vi "Is Express VI.vi"(8 "error in":errorcluster, 11 "VI Reference":refnum<vi>) -> (0 "error out":errorcluster, 1 "Is Instance":bool, 2 "Is Express VI":bool, 3 "Display Name":string)   [LabVIEW 2020, in "Peek Window.lvlib"]
uses:
  Peek Window.lvlib
  8898ce48-ddb9-4dd9-ab7b-7e2c6aebdd87.vi
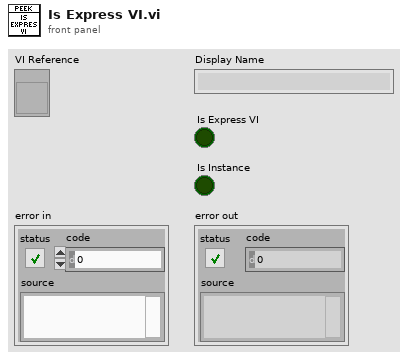
[diagram p1: front panel]
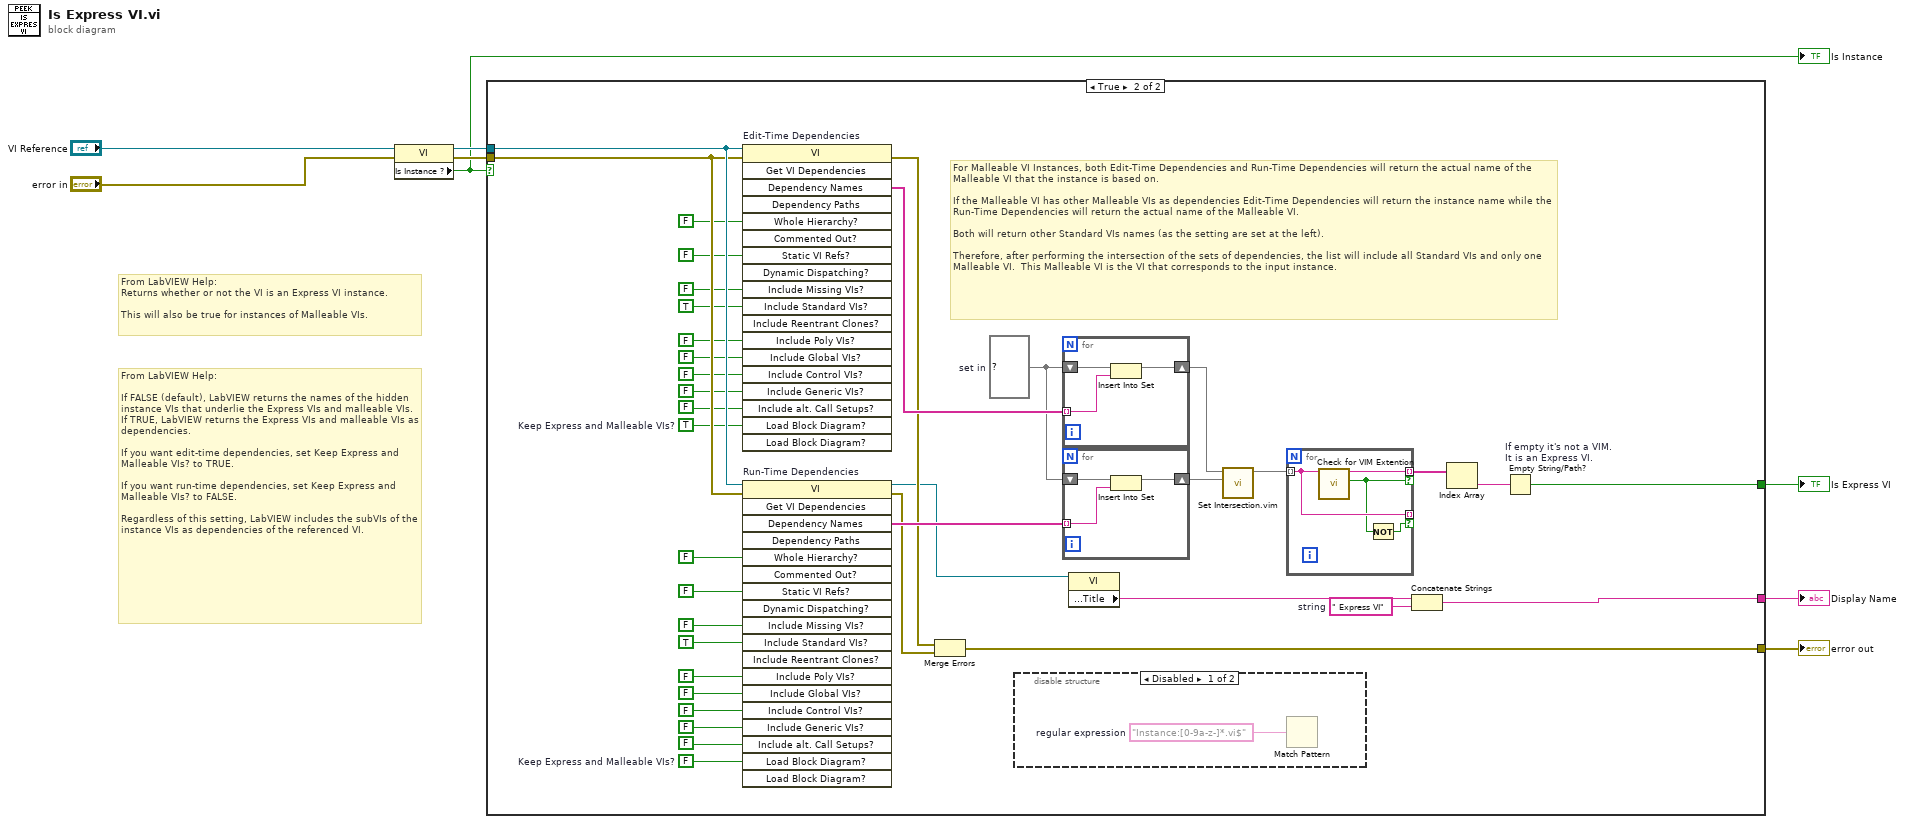
[diagram p0: block diagram]
diagram:
  # "From LabVIEW Help:\nReturns whether or not the VI is an Express VI instance.\n\nThis will also be true for instances of Malleable VIs."
  # "From LabVIEW Help:\n\nIf FALSE (default), LabVIEW returns the names of the hidden instance VIs that underlie the Express VIs and malleable VIs. If TRUE, LabVIEW returns the Express VIs and malleable VIs as dependencies.\n\nIf you want edit-time dependencies, set Keep Express and Malleable VIs? to TRUE. \n\nIf you want run-time dependencies, set Keep Express and Malleable VIs? to FALSE. \n\nRegardless of this setting, LabVIEW includes the subVIs of the instance VIs as dependencies of the referenced VI."
  n1 = property class="VI"(reference="VI Reference", error in="error in") -> (reference out=w8:refnum<vi>, error out=w7:errorcluster, "Is Instance ?"=w3:bool)
  "Is Instance" <- w3
  n2 = case shown="True" w3 {
    tunnel: w8 -> [_ w47]
    tunnel: w7 -> [w9 w45]
    tunnel: [w9 w44] -> w6
    tunnel: [_ w14] -> w2
    tunnel: [_ w11] -> w1
    frame False {
    }
    frame True {
      w10 = " Express VI"  # string
      w19 = set{string} {}  # set in
      w24 = FALSE  # Keep Express and Malleable VIs?
      w43 = TRUE  # Keep Express and Malleable VIs?
      # "For Malleable VI Instances, both Edit-Time Dependencies and Run-Time Dependencies will return the actual name of the Malleable VI that the instance is based on.  \n\nIf the Malleable VI has other Malleable VIs as dependencies Edit-Time Dependencies will return the instance name while the Run-Time Dependencies will return the actual name of the Malleable VI.\n\nBoth will return other Standard VIs names (as the setting are set at the left).\n\nTherefore, after performing the intersection of the sets of dependencies, the list will include all Standard VIs and only one Malleable VI.  This Malleable VI is the VI that corresponds to the input instance."
      n3 = invoke on="Edit-Time Dependencies" class="VI" method="Get VI Dependencies"(reference=w47, error in=w45, "Whole Hierarchy?"=FALSE, "Static VI Refs?"=FALSE, "Include Missing VIs?"=FALSE, "Include Standard VIs?"=TRUE, "Include Poly VIs?"=FALSE, "Include Global VIs?"=FALSE, "Include Control VIs?"=FALSE, "Include Generic VIs?"=FALSE, "Include alt. Call Setups?"=FALSE, "Load Block Diagram?"=w43) -> (error out=w16:errorcluster, "Dependency Names"=w23:string[])  [unwired: 7 in, 17 out]
      n4 = invoke on="Run-Time Dependencies" class="VI" method="Get VI Dependencies"(reference=w47, error in=w45, "Whole Hierarchy?"=FALSE, "Static VI Refs?"=FALSE, "Include Missing VIs?"=FALSE, "Include Standard VIs?"=TRUE, "Include Poly VIs?"=FALSE, "Include Global VIs?"=FALSE, "Include Control VIs?"=FALSE, "Include Generic VIs?"=FALSE, "Include alt. Call Setups?"=FALSE, "Load Block Diagram?"=w24) -> (reference out=w13:refnum<vi>, error out=w15:errorcluster, "Dependency Names"=w18:string[])  [unwired: 7 in, 16 out]
      n5 = Merge Errors(w16, w15) -> (w44:errorcluster)
      n6 = disable-structure shown="Disabled" {
        frame Disabled {
          w48 = "Instance:[0-9a-z-]*.vi$"  # regular expression
          n7 = Match Pattern(regular expression=w48) -> ()  [unwired: 2 in, 4 out]
        }
        frame Enabled {
        }
      }
      n8 = for {
        shift-right: [w51] -> w22
        shift-left: w19 -> [w50]
        tunnel: w23 -> [w49] mode=indexing
        n9 = Insert Into Set(10:w49, 11:w50) -> (3:w51:set{string})  [unwired: 1 out]
      }
      n10 = for {
        shift-right: [w54] -> w17
        shift-left: w19 -> [w53]
        tunnel: w18 -> [w52] mode=indexing
        n11 = Insert Into Set(10:w52, 11:w53) -> (3:w54:set{string})  [unwired: 1 out]
      }
      n12 = property class="VI"(reference=w13) -> ("Front Panel.Title"=w12:string)  [unwired: 1 in, 2 out]
      n13 = call "Set Intersection.vim"("set 2"=w17, "set 1"=w22) -> ("intersection"=w21:set{string})  [unwired: 9 in]
      n14 = for {
        tunnel: w21 -> [w57] mode=indexing
        tunnel: [w58] -> w20 mode=indexing if=w56
        tunnel: [w57] -> _ mode=indexing if=w55
        n15 = call "Check for VIM Extention.vi"("VI Name in"=w57) -> ("Is a Malleable VI"=w56:bool, "VI Name out"=w58:string)  [unwired: 9 in]
        n16 = Not(x=w56) -> (.not. x?=w55:bool)
      }
      n17 = Concatenate Strings(w12, w10) -> (w11:string)
      n18 = Index Array(array=w20) -> (element=w46:string)  [unwired: 1 in]
      n19 = Empty String/Path? "If empty it's not a VIM.\nIt is an Express VI."(string/path=w46) -> (empty?=w14:bool)
    }
  }
  "error out" <- w6
  "Is Express VI" <- w2
  "Display Name" <- w1
